vi "Post-Uninstall Custom Action.vi"(10 "Variant":variant) -> (0 "error out":errorcluster)   [LabVIEW 2020]
uses:
  <vilib>/zip/NI_Unzip.lvlib
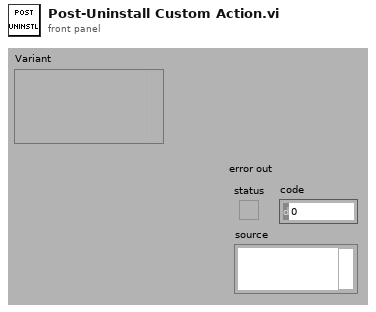
[diagram p1: front panel]
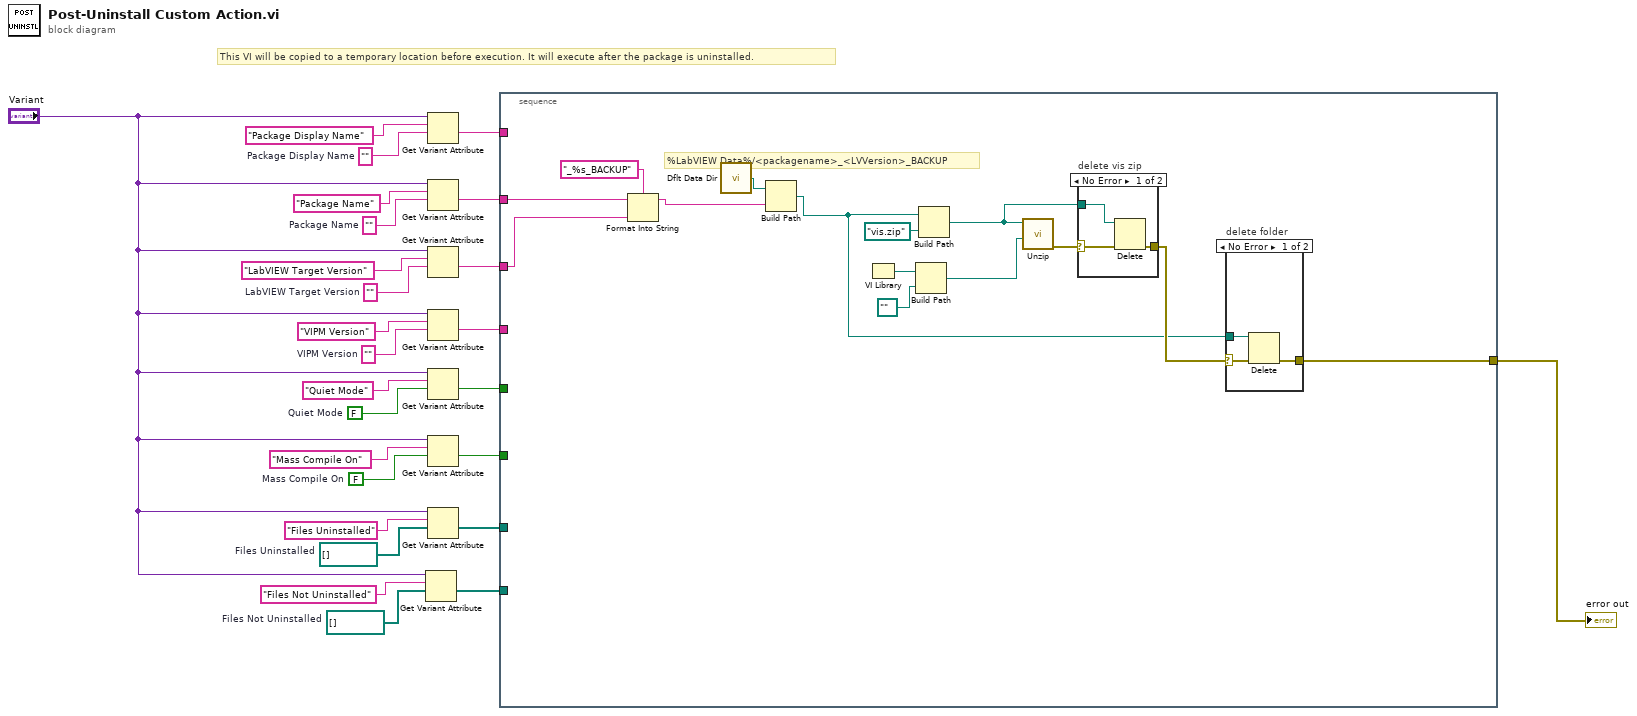
[diagram p0: block diagram]
diagram:
  w2 = path[] []  # Files Not Uninstalled
  w3 = path[] []  # Files Uninstalled
  w9 = FALSE  # Mass Compile On
  w10 = ""  # Package Display Name
  w17 = FALSE  # Quiet Mode
  w20 = ""  # VIPM Version
  w22 = ""  # LabVIEW Target Version
  w24 = ""  # Package Name
  # "This VI will be copied to a temporary location before execution. It will execute after the package is uninstalled."
  n1 = Get Variant Attribute(Variant="Variant", name="Files Not Uninstalled", default value (empty Variant)=w2) -> (value=w7:path[])  [unwired: 1 in, 3 out]
  n2 = Get Variant Attribute(Variant="Variant", name="Package Display Name", default value (empty Variant)=w10) -> (value=w16:string)  [unwired: 1 in, 3 out]
  n3 = Get Variant Attribute(Variant="Variant", name="Package Name", default value (empty Variant)=w24) -> (value=w15:string)  [unwired: 1 in, 3 out]
  n4 = Get Variant Attribute(Variant="Variant", name="LabVIEW Target Version", default value (empty Variant)=w22) -> (value=w14:string)  [unwired: 1 in, 3 out]
  n5 = Get Variant Attribute(Variant="Variant", name="VIPM Version", default value (empty Variant)=w20) -> (value=w13:string)  [unwired: 1 in, 3 out]
  n6 = Get Variant Attribute(Variant="Variant", name="Quiet Mode", default value (empty Variant)=w17) -> (value=w12:bool)  [unwired: 1 in, 3 out]
  n7 = Get Variant Attribute(Variant="Variant", name="Mass Compile On", default value (empty Variant)=w9) -> (value=w11:bool)  [unwired: 1 in, 3 out]
  n8 = Get Variant Attribute(Variant="Variant", name="Files Uninstalled", default value (empty Variant)=w3) -> (value=w6:path[])  [unwired: 1 in, 3 out]
  n9 = stacked-sequence {
    tunnel: w16 -> [_]
    tunnel: w15 -> [w37]
    tunnel: w14 -> [w27]
    tunnel: w13 -> [_]
    tunnel: w12 -> [_]
    tunnel: w11 -> [_]
    tunnel: w6 -> [_]
    tunnel: w7 -> [_]
    tunnel: [w28] -> w1
    frame #0 {
      # "%LabVIEW Data%/<packagename>_<LVVersion>_BACKUP"
      n10 = Format Into String(format string="_%s_BACKUP", initial string=w37, w27) -> (resulting string=w38:string)  [unwired: 1 in, 1 out]
      n11 = call <vilib>:"Dflt Data Dir.vi"() -> ("App:Default Data Directory"=w40:path)
      n12 = Build Path(base path=w40, name or relative path=w38) -> (appended path=w29:path)
      n13 = VI Library() -> (path=w34:path)
      n14 = Build Path(base path=w34, name or relative path=path "..") -> (appended path=w35:path)
      n15 = Build Path(base path=w29, name or relative path=path "vis.zip") -> (appended path=w30:path)
      n16 = call <vilib>:"Unzip.vi"("Target directory (same as Zip file if empty)"=w35, "Zip file"=w30) -> ("error out"=w33:errorcluster)  [unwired: 7 in, 2 out]
      n17 = case "delete vis zip" shown="No Error" w33 {
        selector: w33 -> [w43 w44]
        tunnel: w30 -> [w42 _]
        tunnel: [w41 w44] -> w32
        frame No Error {
          n18 = Delete(path (use dialog)=w42, error in=w43) -> (error out=w41:errorcluster)  [unwired: 3 in, 2 out]
        }
        frame Error {
        }
      }
      n19 = case "delete folder" shown="No Error" w32 {
        selector: w32 -> [w47 w48]
        tunnel: w29 -> [w46 _]
        tunnel: [w45 w48] -> w28
        frame No Error {
          n20 = Delete(path (use dialog)=w46, error in=w47) -> (error out=w45:errorcluster)  [unwired: 3 in, 2 out]
        }
        frame Error {
        }
      }
    }
  }
  "error out" <- w1
